vi "heco top地址获取.vi"() -> ()   [LabVIEW 2020]
uses:
  <vilib>/httpClient/ClientHandle.ctl
  <vilib>/Utility/file.llb/Write Delimited Spreadsheet (string).vi
  <vilib>/httpClient/LabVIEWHTTPClient.lvlib
panel:
  out "URL输出":string
  in  "client handle":T1 caption="客户端句柄"
  in  "error in (no error)":errorcluster caption="错误输入（无错误）"
  out "子字符串之后":string
  out "子字符串之前":string
  out "数组 2":string[](array[string])
  out "地址":string
  out "余额":string
  out "添加的数组":string[](array[string])
  out "数组":string[][](array[string])
  in  "file path (dialog if empty)":path=path "D:/NI 资源包/2-币猎人-事件状态机930/source/网址私钥获取/btc搜寻器/heco前10000账户 .txt" caption="文件路径 （空时为对话框）"
  out "body":string caption="体部"
  out "headers":string caption="头部"
  out "error out":errorcluster caption="错误输出"
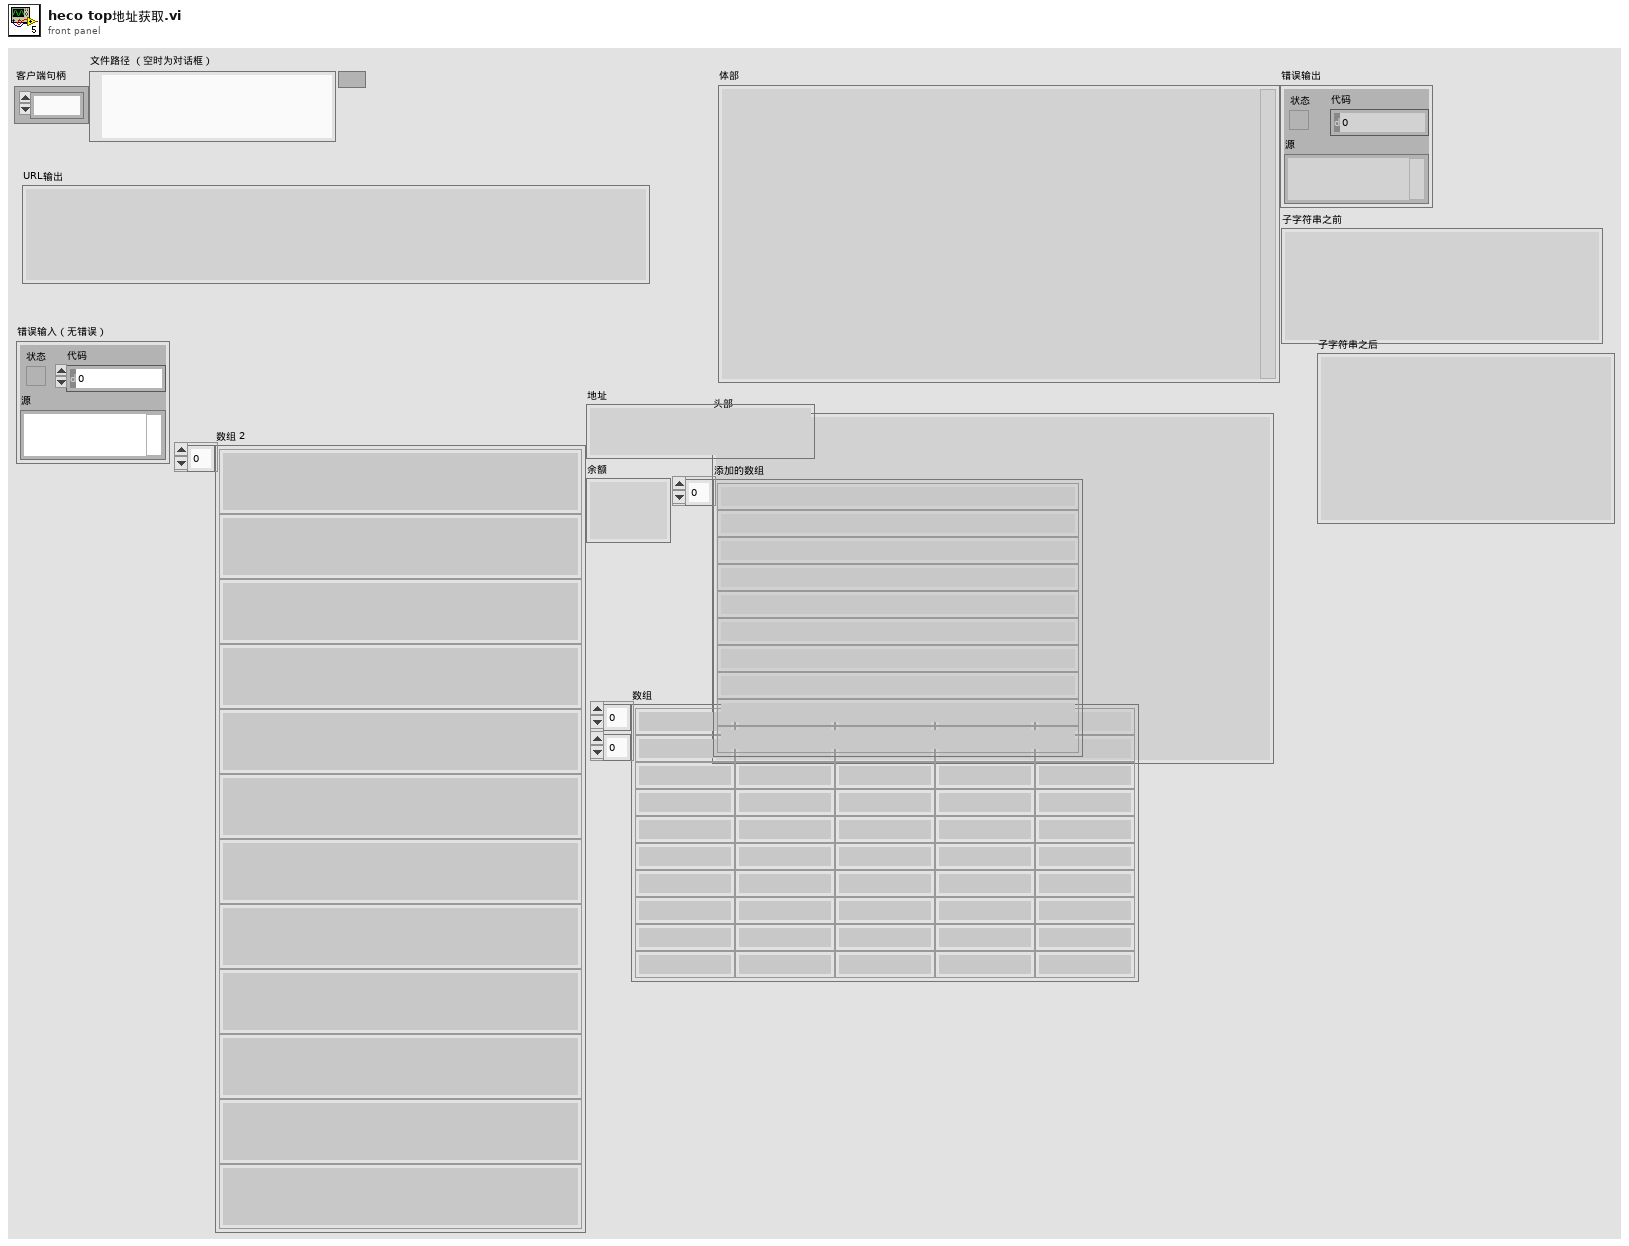
[diagram p1: front panel]
types:
  T1 = typedef "LabVIEWHTTPClient.lvlib/ClientHandle.ctl" = refnum<k1>
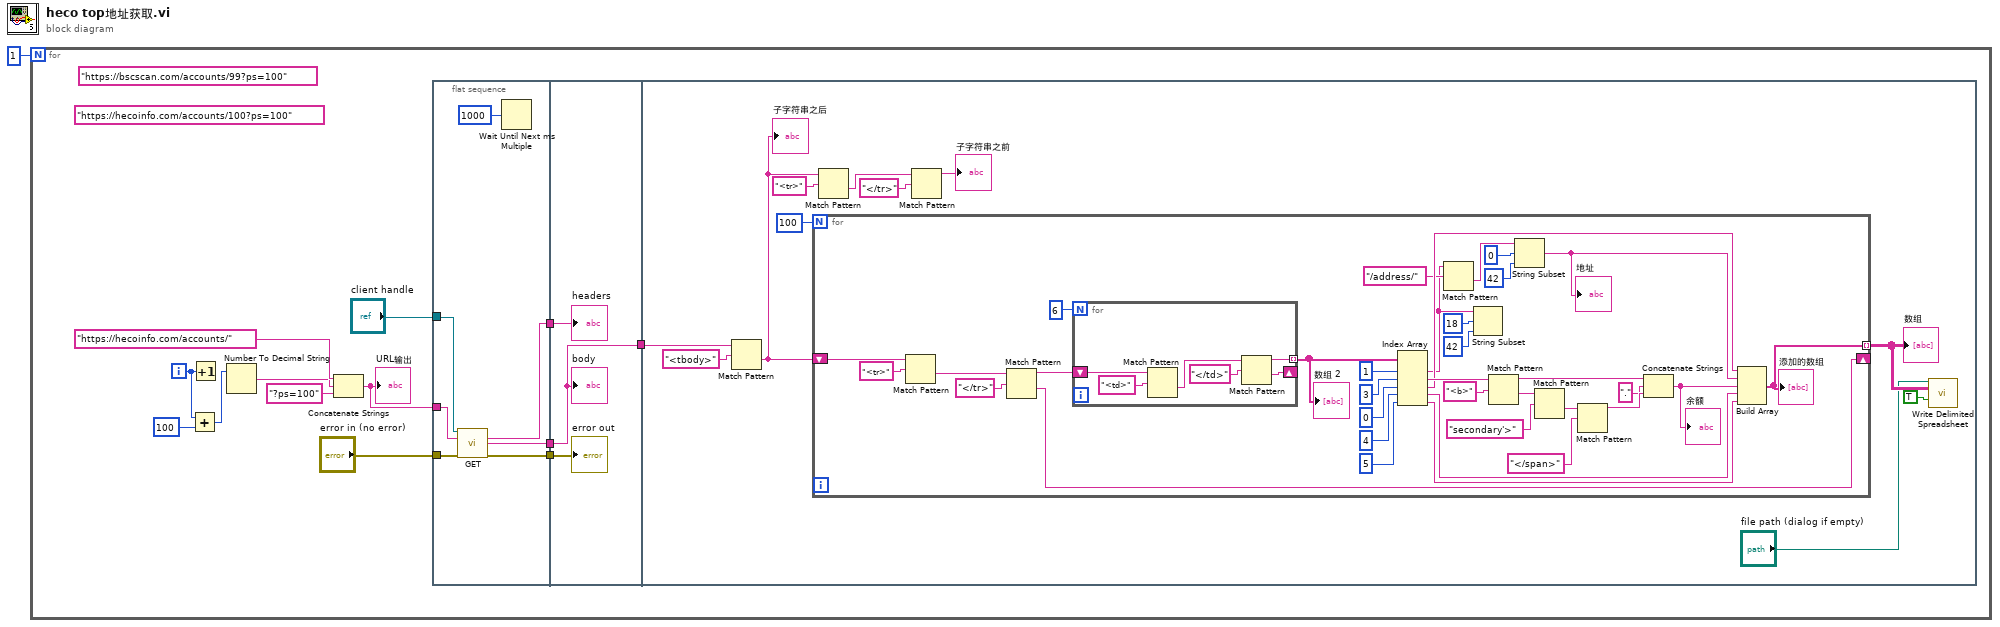
[diagram p0: block diagram]
diagram:
  n1 = for {
    N: 1 -> [_]
    i -> [w4]
    (unwired) "https://hecoinfo.com/accounts/100?ps=100" ("URL输入 2")
    (unwired) "https://bscscan.com/accounts/99?ps=100" ("URL输入 2")
    n2 = Add(x=w4, y=100) -> (x+y=w2:i32)
    n3 = Increment(x=w4) -> ()  [unwired: 1 out]
    n4 = Number To Decimal String(number=w2) -> (decimal integer string=w7:string)  [unwired: 1 in]
    n5 = Concatenate Strings("https://hecoinfo.com/accounts/" ("URL输入 2"), w7, "?ps=100" ("字符串")) -> (w5:string)
    "URL输出" <- w5
    n6 = flat-sequence {
      tunnel: [w18] -> w14
      tunnel: [w17] -> w13
      tunnel: "client handle" -> [w21]
      tunnel: w5 -> [w20]
      tunnel: "error in (no error)" -> [w19]
      tunnel: [w15] -> w12
      tunnel: w14 -> [w24]
      tunnel: w13 -> [w22]
      tunnel: w12 -> [w23]
      tunnel: [w22] -> w11
      tunnel: w11 -> [w35]
      frame #0 {
        n7 = call <vilib>:"GET.vi"("client handle"=w21, "url"=w20, "error in (no error)"=w19) -> ("headers"=w18:string, "body"=w17:string, "error out"=w15:errorcluster)  [unwired: 9 in, 1 out]
        n8 = Wait Until Next ms Multiple(millisecond multiple=u32 1000 ("毫秒倍数")) -> ()  [unwired: 1 out]
      }
      frame #1 {
        "body" <- w22
        "headers" <- w24
        "error out" <- w23
      }
      frame #2 {
        n9 = Match Pattern(string=w35, regular expression="<tbody>") -> (after substring=w28:string)  [unwired: 1 in, 3 out]
        "子字符串之后" <- w28
        n10 = for {
          N: 100 -> [_]
          shift-right: [w66] -> _
          shift-left: w28 -> [w69]
          tunnel: [w42] -> w27 mode=indexing
          n11 = Match Pattern(string=w69, regular expression="<tr>") -> (after substring=w68:string)  [unwired: 1 in, 3 out]
          n12 = Match Pattern(string=w68, regular expression="</tr>" ("正则表达式")) -> (before substring=w43:string, after substring=w66:string)  [unwired: 1 in, 2 out]
          n13 = for {
            N: 6 -> [_]
            shift-right: [w72] -> _
            shift-left: w43 -> [w73]
            tunnel: [w71] -> w64 mode=indexing
            n14 = Match Pattern(string=w73, regular expression="<td>" ("正则表达式")) -> (after substring=w75:string)  [unwired: 1 in, 3 out]
            n15 = Match Pattern(string=w75, regular expression="</td>" ("正则表达式")) -> (before substring=w71:string, after substring=w72:string)  [unwired: 1 in, 2 out]
          }
          "数组 2" <- w64
          n16 = Index Array(array=w64, index #1=1 ("索引"), index #2=3 ("索引"), index #3=0 ("索引"), index #4=4 ("索引"), index #5=5 ("索引")) -> (element #1=w37:string, element #2=w59:string, element #3=w49:string, element #4=w45:string, element #5=w44:string)
          n17 = Match Pattern(string=w37, regular expression="/address/" ("正则表达式")) -> (after substring=w39:string)  [unwired: 1 in, 3 out]
          n18 = String Subset(string=w37, offset (0)=18 ("偏移量(0)"), length (rest)=42 ("长度（剩余）")) -> ()  [unwired: 1 out]
          n19 = Match Pattern(string=w59, regular expression="<b>" ("正则表达式")) -> (before substring=w53:string, after substring=w57:string)  [unwired: 1 in, 2 out]
          n20 = String Subset(string=w39, offset (0)=0 ("偏移量(0)"), length (rest)=42 ("长度（剩余）")) -> (substring=w36:string)
          "地址" <- w36
          n21 = Match Pattern(string=w57, regular expression="secondary'>" ("正则表达式")) -> (after substring=w55:string)  [unwired: 1 in, 3 out]
          n22 = Match Pattern(string=w55, regular expression="</span>" ("正则表达式")) -> (before substring=w52:string)  [unwired: 1 in, 3 out]
          n23 = Concatenate Strings(w53, "." ("字符串"), w52) -> (w48:string)
          "余额" <- w48
          n24 = Build Array(w49, w36, w48, w45, w44) -> (w42:string[])
          "添加的数组" <- w42
        }
        "数组" <- w27
        n25 = Match Pattern(string=w28, regular expression="<tr>") -> (after substring=w32:string)  [unwired: 1 in, 3 out]
        n26 = Match Pattern(string=w32, regular expression="</tr>" ("正则表达式")) -> (before substring=→"子字符串之前":string)  [unwired: 1 in, 3 out]
        n27 = call-poly <vilib>:"Write Delimited Spreadsheet.vi"("file path (dialog if empty)"="file path (dialog if empty)", "2D data"=w27, "append to file? (new file:F)"=TRUE) -> ()  [unwired: 11 in, 2 out]
      }
    }
  }
